vi "CMN_SendMail.vi"(5 "file with text":path, 7 "tmp dir":path, 9 "body":string, 10 "subject":string, 11 "address":string) -> ()   [LabVIEW 2016]
doc: "Will send an e-mail to the specified address. The subject must be specified on the subject input.\nFor the body:\n- If a file is specified, that one will be used.\n- If no file is provided, then it will use the \"body\" entry. If a tmp dir is provided, it will use that one for creating a temporary file with the text. If no tmp dir is provided, it will try using the current dir. The temmporary file will be deleted after sending the mail"
panel:
  out "standard error":string
  out "standard output":string
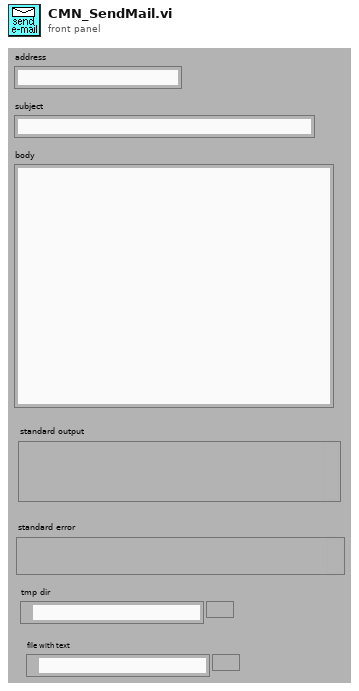
[diagram p1: front panel]
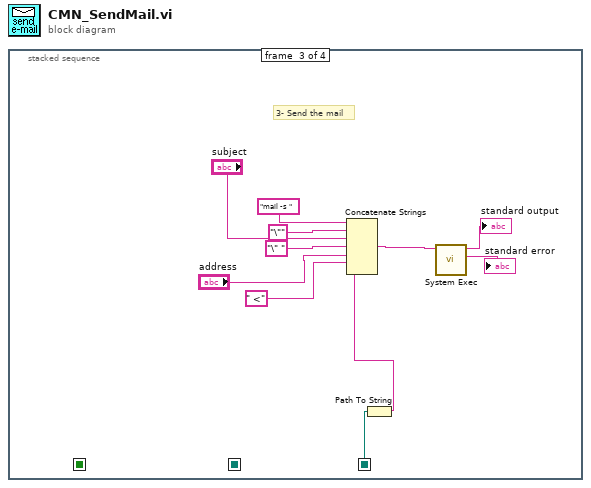
[diagram p0: block diagram]
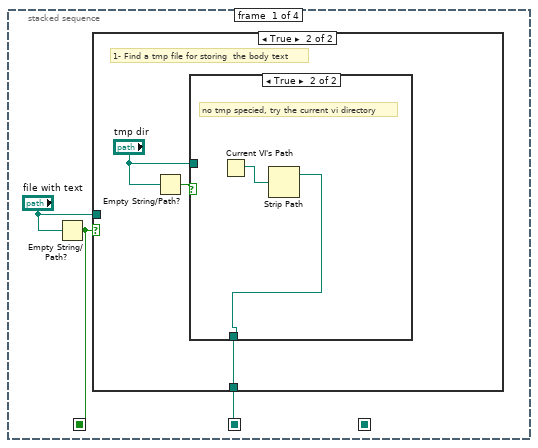
[diagram p2: hidden frame]
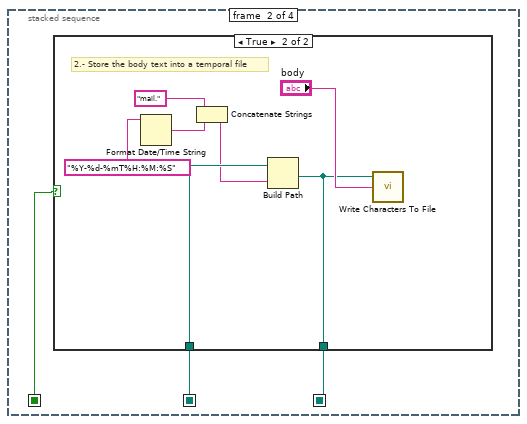
[diagram p5: hidden frame]
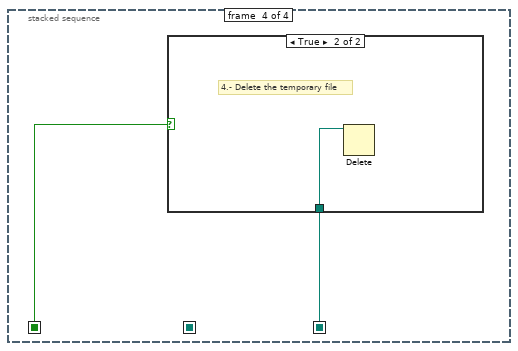
[diagram p7: hidden frame]
diagram:
  n1 = stacked-sequence {
    seq-local: [w3 _ _ _] -> [_ w13 _ _]
    seq-local: [_ w12 _ _] -> [_ _ w24 w34]
    seq-local: [w2 _ _ _] -> [_ w11 _ w33]
    frame #0 {
      n2 = Empty String/Path?(string/path="file with text") -> (empty?=w2:bool)
      n3 = case shown="True" w2 {
        tunnel: [w4 w5] -> w3
        tunnel: "file with text" -> [w4 _]
        frame False {
          # "will use the provided file for the text"
        }
        frame True {
          # "1- Find a tmp file for storing  the body text"
          n4 = Empty String/Path?(string/path="tmp dir") -> (empty?=w7:bool)
          n5 = case shown="True" w7 {
            tunnel: "tmp dir" -> [w8 _]
            tunnel: [w8 w9] -> w5
            frame False {
              # "tmp dir specified, use it"
            }
            frame True {
              # "no tmp specied, try the current vi directory"
              n6 = Current VI's Path() -> (path=w10:path)
              n7 = Strip Path(path=w10) -> (stripped path=w9:path)  [unwired: 1 out]
            }
          }
        }
      }
    }
    frame #1 {
      n8 = case shown="True" w11 {
        tunnel: w13 -> [w14 w19]
        tunnel: [w14 w16] -> w12
        frame False {
          # "will use the provided file"
        }
        frame True {
          # "2.- Store the body text into a temporal file"
          n9 = Format Date/Time String(time format string (%c)="%Y-%d-%mT%H:%M:%S") -> (date/time string=w21:string)  [unwired: 2 out]
          n10 = Concatenate Strings("mail.", w21) -> (w18:string)
          n11 = Build Path(base path=w19, name or relative path=w18) -> (appended path=w16:path)
          n12 = call <vilib>:"Write Characters To File.vi"("character string"="body", "file path (dialog if empty)"=w16) -> ()  [unwired: 1 in, 3 out]
        }
      }
    }
    frame #2 {
      # "3- Send the mail"
      n13 = Path To String(path=w24) -> (string=w23:string)
      n14 = Concatenate Strings("mail -s " ("command line"), "\"" ("string"), "subject", "\" " ("string"), "address", " <" ("string"), w23) -> (w22:string)
      n15 = call <vilib>:"System Exec.vi"("command line"=w22) -> ("standard error"=→"standard error":string, "standard output"=→"standard output":string)  [unwired: 5 in, 4 out]
    }
    frame #3 {
      n16 = case shown="True" w33 {
        tunnel: w34 -> [_ w35]
        frame False {
          # "do not delete the provided file"
        }
        frame True {
          # "4.- Delete the temporary file"
          n17 = Delete(path (use dialog)=w35) -> ()  [unwired: 1 in, 6 out]
        }
      }
    }
  }
